vi "Convert Register Address To Array.vi"(1 "Register Address Size":T1, 2 "Register":u32) -> (0 "Register Address Array":u8[](array[numeric]))   [LabVIEW 2020, in "lv_i2c_hal.lvlib" / "I2C.lvclass"]
uses:
  I2C.lvclass
  Register Address Size.ctl
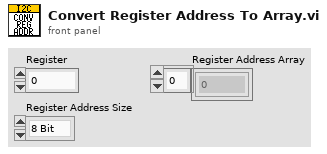
[diagram p1: front panel]
types:
  T1 = typedef "lv_i2c_hal.lvlib/I2C.lvclass/Register Address Size.ctl" = enum16{"8 Bit", "16 Bit", "24 Bit", "32 Bit"}
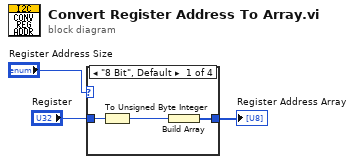
[diagram p0: block diagram]
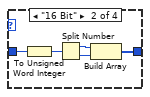
[diagram p2: hidden frame]
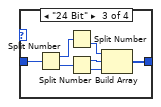
[diagram p3: hidden frame]
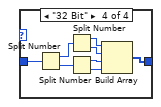
[diagram p4: hidden frame]
diagram:
  n1 = case shown="\"8 Bit\", Default" "Register Address Size" {
    tunnel: [w5 w8 w12 w19] -> w1
    tunnel: "Register" -> [w4 w7 w18 w26]
    frame "8 Bit", Default {
      n2 = To Unsigned Byte Integer(number=w4) -> (unsigned 8bit integer=w6:u8)
      n3 = Build Array(w6) -> (w5:u8[])
    }
    frame "16 Bit" {
      n4 = To Unsigned Word Integer(number=w7) -> (unsigned 16bit integer=w11:u16)
      n5 = Split Number(x=w11) -> (hi(x)=w10:u8, lo(x)=w9:u8)
      n6 = Build Array(w10, w9) -> (w8:u8[])
    }
    frame "24 Bit" {
      n7 = Split Number(x=w18) -> (hi(x)=w17:u16, lo(x)=w16:u16)
      n8 = Split Number(x=w17) -> (lo(x)=w15:u8)  [unwired: 1 out]
      n9 = Split Number(x=w16) -> (hi(x)=w14:u8, lo(x)=w13:u8)
      n10 = Build Array(w15, w14, w13) -> (w12:u8[])
    }
    frame "32 Bit" {
      n11 = Split Number(x=w26) -> (hi(x)=w25:u16, lo(x)=w24:u16)
      n12 = Split Number(x=w25) -> (hi(x)=w23:u8, lo(x)=w22:u8)
      n13 = Split Number(x=w24) -> (hi(x)=w21:u8, lo(x)=w20:u8)
      n14 = Build Array(w23, w22, w21, w20) -> (w19:u8[])
    }
  }
  "Register Address Array" <- w1
